vi "ConfigDa.vi"(0 "Pump_1AI_1DO_2DI in":refnum<class "PM_Group.lvclass">, 11 "error in (no error)":errorcluster) -> (4 "Pump_1AI_1DO_2DI out":refnum<class "PM_Group.lvclass">, 15 "error out":errorcluster)   [LabVIEW 2019, in "PM_Group.lvclass"]
uses:
  PM_Group.lvclass
  D:/GIT H4000/H4000/src/Proccess_class/Proccess.lvclass
  Sig_DA_class/Sig_DA.lvclass
  Proccess_class/Proccess.lvclass/Proccess.ctl
  PM_Group.lvclass/PM_Group.ctl
  Proccess_class/Proccess.lvclass
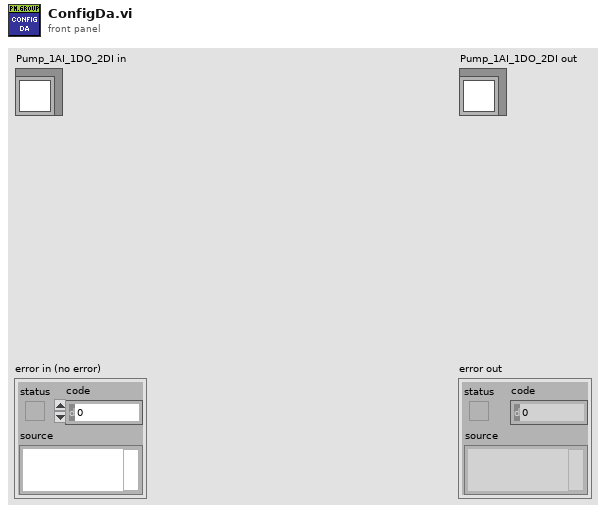
[diagram p1: front panel]
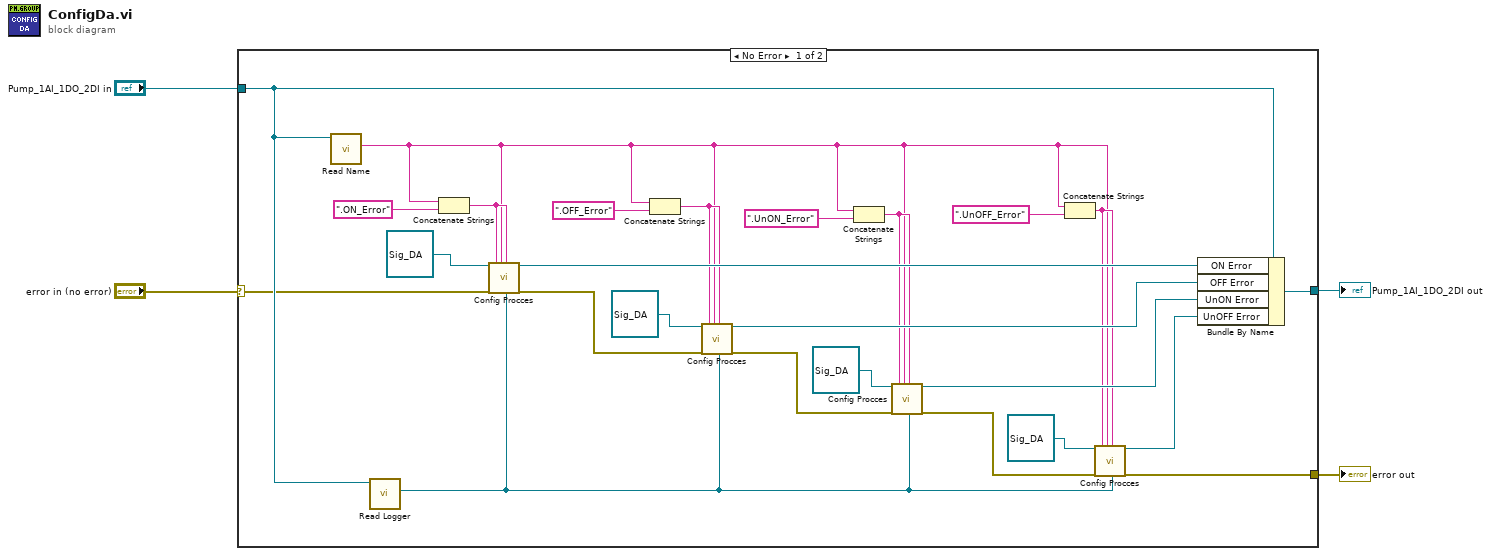
[diagram p0: block diagram]
diagram:
  n1 = case shown="No Error" "error in (no error)" {
    selector: "error in (no error)" -> [w6 w31]
    tunnel: [w5 w31] -> w3
    tunnel: [w29 w30] -> w1
    tunnel: "Pump_1AI_1DO_2DI in" -> [w19 w30]
    frame No Error {
      n2 = call "Read Name.vi"("Proccess in"=w19) -> ("Name"=w10:string)  [unwired: 10 in]
      n3 = call "Read Logger.vi"("Proccess in"=w19) -> ("Logger"=w20:refnum<class "Logger.lvclass">)  [unwired: 10 in]
      n4 = Concatenate Strings(w10, ".ON_Error" ("string")) -> (w17:string)
      n5 = call "Config Procces.vi"("reference in"=refnum<class "Sig_DA.lvclass"> refnum ("Sig_DA"), "error in (no error)"=w6, "Name"=w17, "ParentName"=w10, "Description"=w17, "Logger"=w20) -> ("reference out"=w28:refnum<class "Sig_DA.lvclass">, "error out"=w9:errorcluster)  [unwired: 12 in]
      n6 = Concatenate Strings(w10, ".OFF_Error" ("string")) -> (w15:string)
      n7 = call "Config Procces.vi"("reference in"=refnum<class "Sig_DA.lvclass"> refnum ("Sig_DA"), "error in (no error)"=w9, "Name"=w15, "ParentName"=w10, "Description"=w15, "Logger"=w20) -> ("reference out"=w27:refnum<class "Sig_DA.lvclass">, "error out"=w8:errorcluster)  [unwired: 12 in]
      n8 = Concatenate Strings(w10, ".UnON_Error" ("string")) -> (w13:string)
      n9 = call "Config Procces.vi"("reference in"=refnum<class "Sig_DA.lvclass"> refnum ("Sig_DA"), "error in (no error)"=w8, "Name"=w13, "ParentName"=w10, "Description"=w13, "Logger"=w20) -> ("reference out"=w26:refnum<class "Sig_DA.lvclass">, "error out"=w7:errorcluster)  [unwired: 12 in]
      n10 = Concatenate Strings(w10, ".UnOFF_Error" ("string")) -> (w11:string)
      n11 = call "Config Procces.vi"("reference in"=refnum<class "Sig_DA.lvclass"> refnum ("Sig_DA"), "error in (no error)"=w7, "Name"=w11, "ParentName"=w10, "Description"=w11, "Logger"=w20) -> ("reference out"=w25:refnum<class "Sig_DA.lvclass">, "error out"=w5:errorcluster)  [unwired: 12 in]
      n12 = Bundle By Name(cluster=w19, "ON Error"=w28, "OFF Error"=w27, "UnON Error"=w26, "UnOFF Error"=w25) -> (w29:refnum<class "PM_Group.lvclass">)
    }
    frame Error {
    }
  }
  "error out" <- w3
  "Pump_1AI_1DO_2DI out" <- w1
